vi "Gyro Read Velocity.vi"(8 "error in (no error)":errorcluster, 11 "FPGA Information In":T2) -> (0 "error out":errorcluster, 2 "Gyro Velocities":T1, 3 "FPGA Information Out":T2)   [LabVIEW 2012]
uses:
  <vilib>/IEDriver/SPIandI2C/Host/I2C/I2C Host.lvlib
panel:
  out "Read Data":u8[](array[numeric])
  in  "Timeout (1 s)":u8=1
  in  "Write Data":u8[](array[numeric])=[29] format="%.0x"
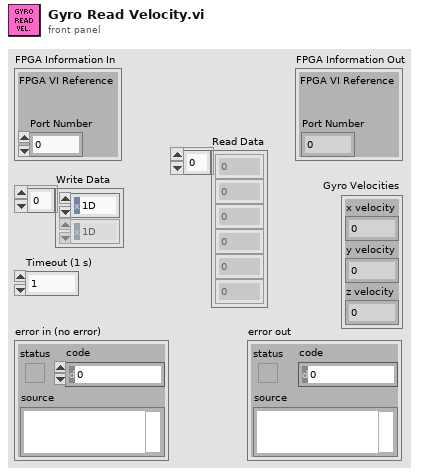
[diagram p1: front panel]
types:
  T1 = cluster{"x velocity":dbl, "y velocity":dbl, "z velocity":dbl}
  T2 = cluster{"FPGA VI Reference":refnum<k20>, "Port Number":u8}
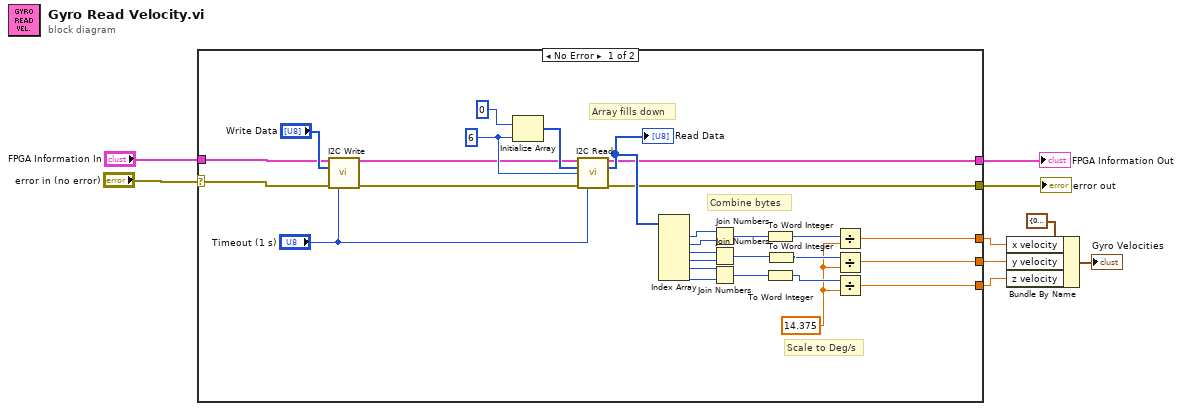
[diagram p0: block diagram]
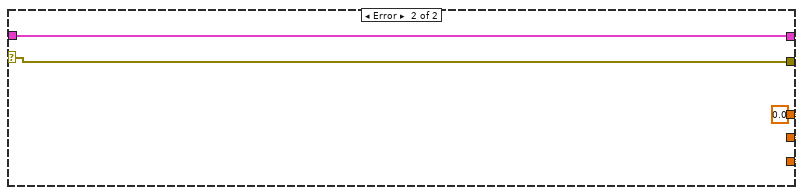
[diagram p2: hidden frame]
diagram:
  n1 = case shown="No Error" "error in (no error)" {
    selector: "error in (no error)" -> [w15 w39]
    tunnel: "FPGA Information In" -> [w26 w40]
    tunnel: [w17 w40] -> w8
    tunnel: [w16 w39] -> w7
    tunnel: [w14 w38] -> w4
    tunnel: [w13 w38] -> w3
    tunnel: [w12 w38] -> w2
    frame No Error {
      w18 = 14.375
      w35 = u16 6 ("Number of Bytes to Read")
      # "Scale to Deg/s"
      # "Combine bytes"
      # "Array fills down"
      n2 = call <vilib>:"I2C Write.vi"("FPGA Information In"=w26, "Data"="Write Data", "error in (no error)"=w15, "Timeout (10 s)"="Timeout (1 s)") -> ("FPGA Information Out"=w11:T2, "error out"=w10:errorcluster)  [unwired: 10 in]
      n3 = Initialize Array(u8 0, w35) -> (w33:u8[])
      n4 = call <vilib>:"I2C Read.vi"("FPGA Information In"=w11, "Input Array"=w33, "Number of Bytes to Read"=w35, "error in (no error)"=w10, "Timeout (10 s)"="Timeout (1 s)") -> ("FPGA Information Out"=w17:T2, "Data"=w32:u8[], "error out"=w16:errorcluster)  [unwired: 8 in]
      "Read Data" <- w32
      n5 = Index Array(array=w32) -> (element #1=w30:u8, element #2=w29:u8, element #3=w28:u8, element #4=w27:u8, element #5=w25:u8, element #6=w24:u8)  [unwired: 6 in]
      n6 = Join Numbers(hi=w30, lo=w29) -> ((hi.lo)=w21:u16)
      n7 = Join Numbers(hi=w28, lo=w27) -> ((hi.lo)=w31:u16)
      n8 = Join Numbers(hi=w25, lo=w24) -> ((hi.lo)=w22:u16)
      n9 = To Word Integer(number=w21) -> (16bit integer=w20:i16)
      n10 = To Word Integer(number=w22) -> (16bit integer=w19:i16)
      n11 = To Word Integer(number=w31) -> (16bit integer=w23:i16)
      n12 = Divide(x=w20, y=w18) -> (x/y=w14:dbl)
      n13 = Divide(x=w23, y=w18) -> (x/y=w13:dbl)
      n14 = Divide(x=w19, y=w18) -> (x/y=w12:dbl)
    }
    frame Error {
      w38 = 0.0
    }
  }
  "error out" <- w7
  "FPGA Information Out" <- w8
  n15 = Bundle By Name(cluster=T1 {"x velocity"=0.0, "y velocity"=0.0, "z velocity"=0.0}, "x velocity"=w4, "y velocity"=w3, "z velocity"=w2) -> (→"Gyro Velocities":T1)
